vi "Clear Faults.vi"(0 "GEA2 Reference In":refnum<k24>, 11 "Error In":errorcluster) -> (2 "Expected Array":string[](array[string]), 3 "Actual Array":string[](array[string]), 4 "GEA2 Reference Out":refnum<k24>, 6 "Pass/Fail?":bool, 8 "Report Text":string, 15 "Error Out":errorcluster)   [LabVIEW 2016, in "Centauro.lvlib"]
doc: "Use this VI to clear all faults (table and sequence)."
uses:
  Projects/Centauro.lvlib
  Q:/Common/DLLs/GEA3/GeaCommunication.dll
  Common/DLLs/GEA3/GeaCommunication.dll
  Common/LabVIEW GEA2 Toolkit/LabVIEW_GEA2_Toolkit.lvlibp/type defs/ERD Write Data In.ctl
  Common/LabVIEW GEA2 Toolkit/LabVIEW_GEA2_Toolkit.lvlibp/type defs/Data Type.ctl
  Common/LabVIEW GEA2 Toolkit/LabVIEW_GEA2_Toolkit.lvlibp/type defs/Source_Destination.ctl
  Common/LabVIEW GEA2 Toolkit/LabVIEW_GEA2_Toolkit.lvlibp/type defs/ERD Read Data In.ctl
  Common/LabVIEW GEA2 Toolkit/LabVIEW_GEA2_Toolkit.lvlibp
panel:
  in  "Standalone?":bool
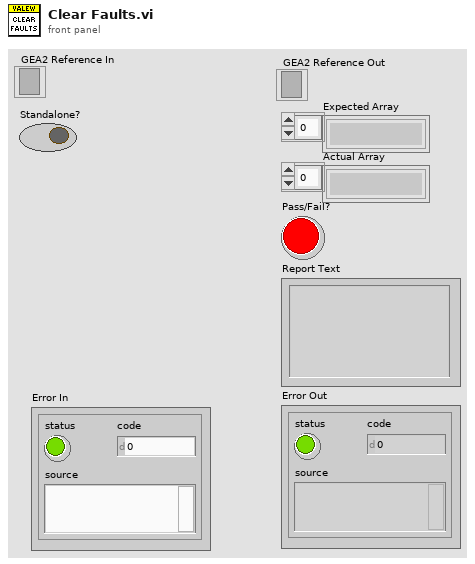
[diagram p1: front panel]
types:
  T1 = typedef "LabVIEW_GEA2_Toolkit.lvlibp/ERD Read Data In.ctl" = cluster{"ERD Number":u16, "Data Type":T2}
  T2 = typedef "LabVIEW_GEA2_Toolkit.lvlibp/Data Type.ctl" = enum16{"string", "boolean", "uint8_t", "uint16_t", "uint32_t", "uint64_t", "int8_t", "int16_t", "int32_t", "int64_t"}
  T3 = typedef "LabVIEW_GEA2_Toolkit.lvlibp/Source_Destination.ctl" = cluster{"Source":u8, "Destination":u8}
  T4 = typedef "LabVIEW_GEA2_Toolkit.lvlibp/ERD Write Data In.ctl" = cluster{"ERD Number":u16, "Data Type":T2, "Data":string}
  T5 = typedef "LabVIEW_GEA2_Toolkit.lvlibp/ERD Read Data Out.ctl" = cluster{"ERD Number":u16, "Data":string}
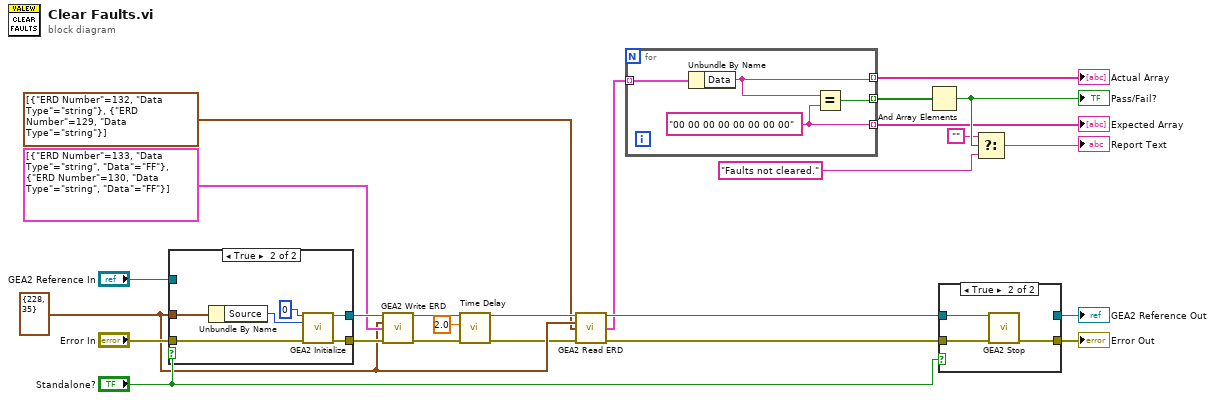
[diagram p0: block diagram]
diagram:
  w14 = T3 {"Source"=228, "Destination"=35} ("GEA Inputs")
  n1 = case shown="True" "Standalone?" {
    tunnel: "Error In" -> [w25 w32]
    tunnel: [w25 w31] -> w18
    tunnel: "GEA2 Reference In" -> [w26 _]
    tunnel: [w26 w30] -> w24
    tunnel: w14 -> [_ w28]
    frame False {
    }
    frame True {
      n2 = Unbundle By Name(w28) -> ("Source"=w29:u8)
      n3 = call "GEA2 Initialize.vi"("Board Index"=0, "Source Address"=w29, "error in"=w32) -> ("GEA2 Reference Out"=w30:refnum<k24>, "error out"=w31:errorcluster)  [unwired: 10 in, 1 out]
    }
  }
  n4 = call "GEA2 Write ERD.vi"("GEA2 Reference In"=w24, "GEA Inputs"=w14, "Write ERD List"=T4[] [{"ERD Number"=133, "Data Type"=enum."string", "Data"="FF"}, {"ERD Number"=130, "Data Type"=enum."string", "Data"="FF"}], "Error In"=w18) -> ("GEA2 Reference Out"=w16:refnum<k24>, "Error Out"=w15:errorcluster)  [unwired: 9 in, 1 out]
  n5 = call "Time Delay"("error in (no error)"=w15, "Delay Time (s)"=2.0) -> ("error out"=w6:errorcluster)  [unwired: 9 in]
  n6 = call "GEA2 Read ERD.vi"("GEA2 Reference In"=w16, "GEA Inputs"=w14, "Read ERD List"=T1[] [{"ERD Number"=132, "Data Type"=enum."string"}, {"ERD Number"=129, "Data Type"=enum."string"}], "Error In"=w6) -> ("GEA2 Reference Out"=w12:refnum<k24>, "ERD Data Out"=w10:T5[], "Error Out"=w11:errorcluster)  [unwired: 8 in, 1 out]
  n7 = for {
    tunnel: w10 -> [w36] mode=indexing
    tunnel: [w35] -> w4 mode=indexing
    tunnel: [w34] -> w2 mode=indexing
    tunnel: [w33] -> w1 mode=indexing
    w34 = "00 00 00 00 00 00 00 00" ("y")
    n8 = Unbundle By Name(w36) -> ("Data"=w33:string)
    n9 = Equal?(x=w33, y=w34) -> (x = y?=w35:bool)
  }
  "Expected Array" <- w2
  "Actual Array" <- w1
  n10 = And Array Elements(Boolean array=w4) -> (logical AND=w9:bool)
  "Pass/Fail?" <- w9
  n11 = case shown="True" "Standalone?" {
    tunnel: w11 -> [w38 w41]
    tunnel: [w38 w40] -> w23
    tunnel: [w37 _] -> w22
    tunnel: w12 -> [w37 w39]
    frame False {
    }
    frame True {
      n12 = call "GEA2 Stop.vi"("GEA2 Reference In"=w39, "Error In"=w41) -> ("Error Out"=w40:errorcluster)  [unwired: 13 in]
    }
  }
  "Error Out" <- w23
  "GEA2 Reference Out" <- w22
  n13 = Select(t="", s=w9, f="Faults not cleared.") -> (s? t:f=→"Report Text":string)
